vi "Override and Call.vi"(8 "error in (no error)":errorcluster, 11 "Parent in":refnum<class "Parent.lvclass">) -> (0 "error out":errorcluster, 3 "Parent out":refnum<class "Parent.lvclass">)   [LabVIEW 2021, in "Parent.lvclass"]
uses:
  Parent.lvclass
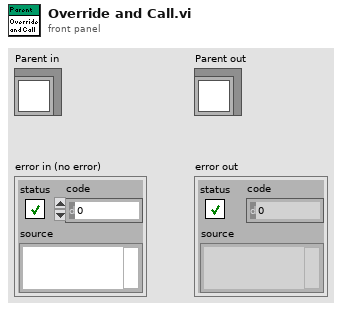
[diagram p1: front panel]
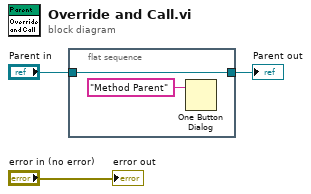
[diagram p0: block diagram]
diagram:
  n1 = flat-sequence {
    tunnel: [w4] -> w2
    tunnel: "Parent in" -> [w4]
    frame #0 {
      n2 = One Button Dialog(message="Method Parent") -> ()  [unwired: 1 in, 1 out]
    }
  }
  "error out" <- "error in (no error)"
  "Parent out" <- w2
